vi "实验第一题.vi"() -> ()   [LabVIEW 2018]
panel:
  out "运行+ 1":dbl
  out "输出":dbl
  in  "输入":dbl
  out "开方":dbl
  in  "数值 7":dbl
  out "数值 6":dbl
  in  "数值 5":dbl
  in  "数值 4":dbl
  in  "数值 3":dbl
  in  "数值 2":dbl
  out "三角形的面积":dbl
  in  "h":dbl
  in  "a":dbl
  out "温度计":dbl(slide) scale=0.0..80.0
  out "液罐":dbl(slide) scale=0.0..9.0
  out "滑动杆":u8(slide) scale=0.0..100.0
  in  "转盘":dbl(knob) scale=0.0..10.0
  in  "旋钮":dbl(knob) scale=0.0..10.0
  out "波形图表":dbl(graph)
  out "布尔":bool
  in  "数值":dbl
  # "前面 板的创建 练习 ：创建并放置多种控件， \n修改它们的大小、 位置、颜色内容量程 等"
  # "求三角形面积"
  # "多个数据求和"
  # "开方"
  # "编写 VI ，进行简单的数学运算：求三角形面积、多个据 的和与开方"
  # "求数学函数，如\n\n3cossinxxxxyxee"
  # "利用局部变量写一个计数器，每当 VI 循环一次，计数器就加一"
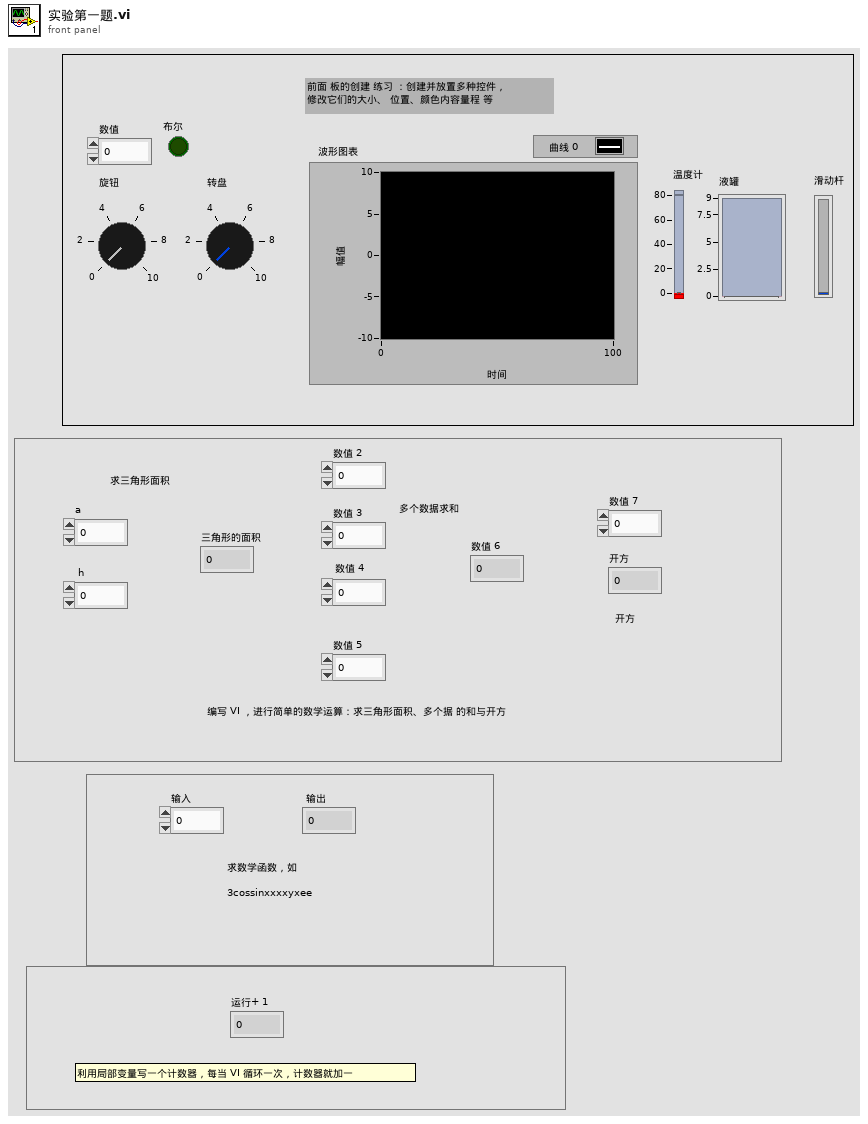
[diagram p1: front panel]
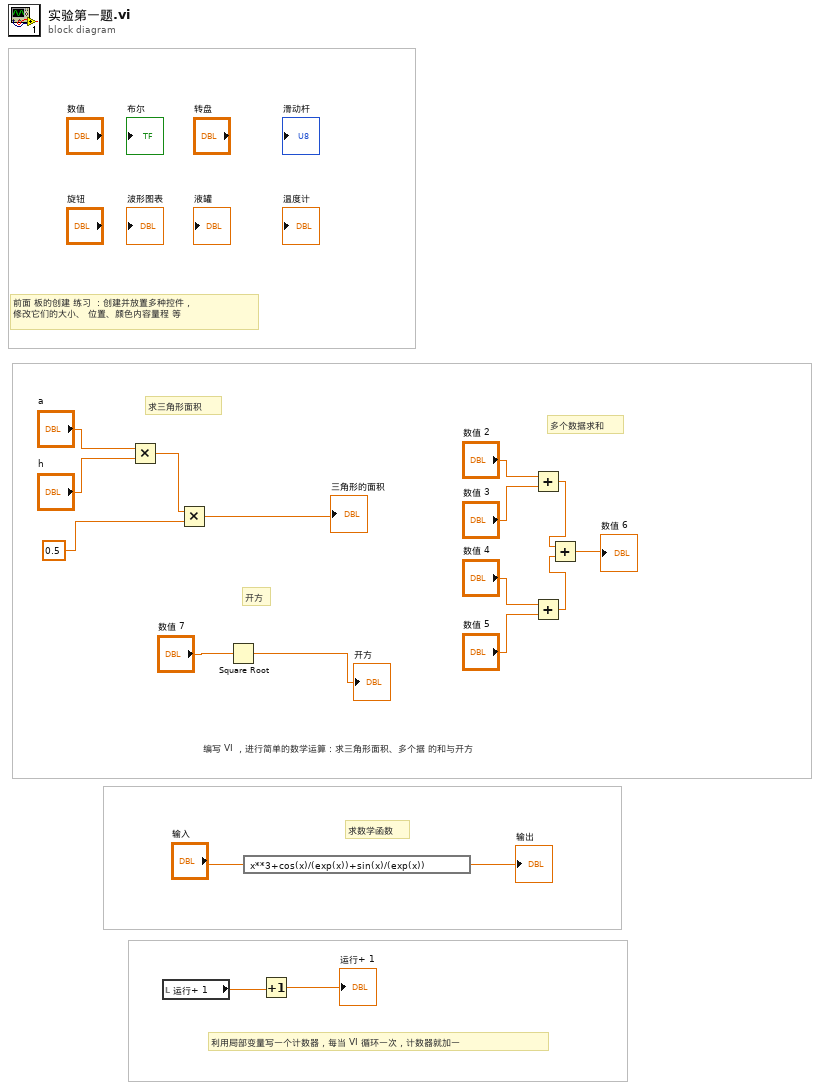
[diagram p0: block diagram]
diagram:
  # "利用局部变量写一个计数器，每当 VI 循环一次，计数器就加一"
  # "求数学函数"
  # "编写 VI ，进行简单的数学运算：求三角形面积、多个据 的和与开方"
  # "开方"
  # "多个数据求和"
  # "求三角形面积"
  # "前面 板的创建 练习 ：创建并放置多种控件， \n修改它们的大小、 位置、颜色内容量程 等"
  n1 = Multiply(x="a", y="h") -> (x*y=w15:dbl)
  n2 = local read "运行+ 1"() -> (w2:dbl)
  n3 = Multiply(x=w15, y=0.5) -> (x*y=→"三角形的面积":dbl)
  n4 = Square Root(x="数值 7") -> (sqrt(x)=→"开方":dbl)
  n5 = expression code="x**3+cos(x)/(exp(x))+sin(x)/(exp(x))" ("表达式节点")("输入") -> (→"输出":dbl)
  n6 = Increment(x=w2) -> (x+1=→"运行+ 1":dbl)
  n7 = Add(x="数值 2", y="数值 3") -> (x+y=w9:dbl)
  n8 = Add(x="数值 4", y="数值 5") -> (x+y=w8:dbl)
  n9 = Add(x=w9, y=w8) -> (x+y=→"数值 6":dbl)
